vi "Set Property.vi"(5 "property value":variant, 7 "property name":string, 8 "error in (no error)":errorcluster, 9 "channel name":string, 10 "group name":string, 11 "File in":refnum<class "File.lvclass">) -> (0 "error out":errorcluster, 1 "channel name out":string, 2 "group name out":string, 3 "File out":refnum<class "File.lvclass">)   [LabVIEW 2016, in "File.lvclass"]
uses:
  File.lvclass
  File.lvclass/File.ctl
  Read tdms stream.vi
  Write tdms stream.vi
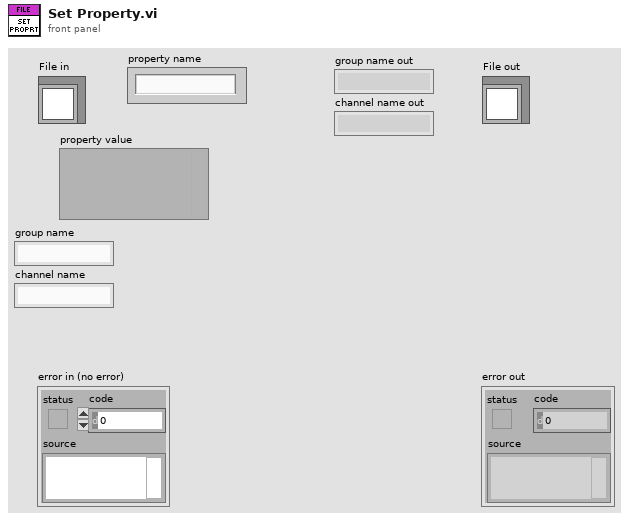
[diagram p1: front panel]
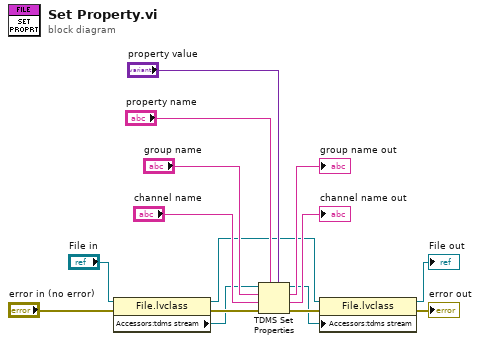
[diagram p0: block diagram]
diagram:
  n1 = property class="File.lvclass"(reference="File in", error in="error in (no error)") -> (reference out=w4:refnum<class "File.lvclass">, error out=w7:errorcluster, "Accessors:tdms stream"=w2:refnum<k34>)
  n2 = TDMS Set Properties(5:"property value", 7:"property name", 8:w7, 9:"channel name", 10:"group name", 11:w2) -> (0:w8:errorcluster, 1:→"channel name out":string, 2:→"group name out":string, 3:w1:refnum<k34>)
  n3 = property class="File.lvclass"(reference=w4, error in=w8, "Accessors:tdms stream"=w1) -> (reference out=→"File out":refnum<class "File.lvclass">, error out=→"error out":errorcluster)
